vi "Write Addr.vi"(8 "error in (no error)":errorcluster, 10 "Addr":refnum<visa-resource-name>, 11 "Lakeshore 218 in":refnum<class "Lakeshore 218.lvclass">) -> (0 "error out":errorcluster, 3 "Lakeshore 218 out":refnum<class "Lakeshore 218.lvclass">)   [LabVIEW 2022 SP3, in "Lakeshore 218.lvclass"]
uses:
  Lakeshore 218.lvclass
  Lakeshore 218.lvclass/Lakeshore 218.ctl
  Temp Control.lvclass
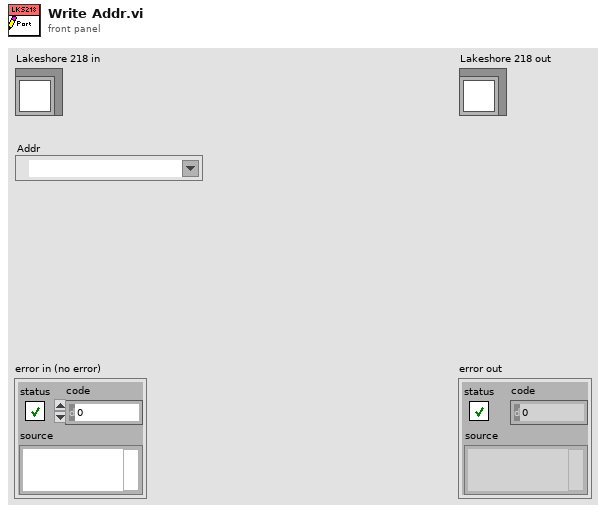
[diagram p1: front panel]
types:
  T1 = typedef "Lakeshore 218.lvclass/Lakeshore 218 cluster Settings.ctl" = cluster{"Port":refnum<visa-resource-name>, "Channel Names":string[], "Ch Enable":bool[]}
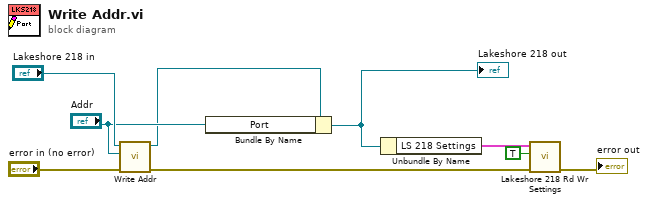
[diagram p0: block diagram]
diagram:
  n1 = call-parent "Write Addr.vi"("error in (no error)"="error in (no error)", "Addr"="Addr", "Temp Control in"="Lakeshore 218 in") -> ("error out"=w5:errorcluster, "Temp Control out"=w6:refnum<class "Lakeshore 218.lvclass">)  [unwired: 7 in]
  n2 = Bundle By Name(cluster=w6, "Port"="Addr") -> (w4:refnum<class "Lakeshore 218.lvclass">)
  "Lakeshore 218 out" <- w4
  n3 = Unbundle By Name(w4) -> ("LS 218 Settings"=w3:T1)
  n4 = call "Lakeshore 218 Rd Wr Settings.vi"("error in (no error)"=w5, "Write? (F:Read)"=TRUE, "LS 218 Settings"=w3) -> ("error out"=→"error out":errorcluster)  [unwired: 7 in, 1 out]
